vi "LVJSON Dump.vi"(4 "PPIsValue? (F)":bool, 6 "PPIndent (0)":i32, 8 "error in (no error)":errorcluster, 10 "Pretty Print? (F)":bool, 11 "Root Element in":T1) -> (0 "error out":errorcluster, 2 "Key":string, 3 "JSON out":string)   [LabVIEW 2018, in "labview_json.lvlib"]
uses:
  labview_json.lvlib
  Element Type.ctl
  Element.ctl
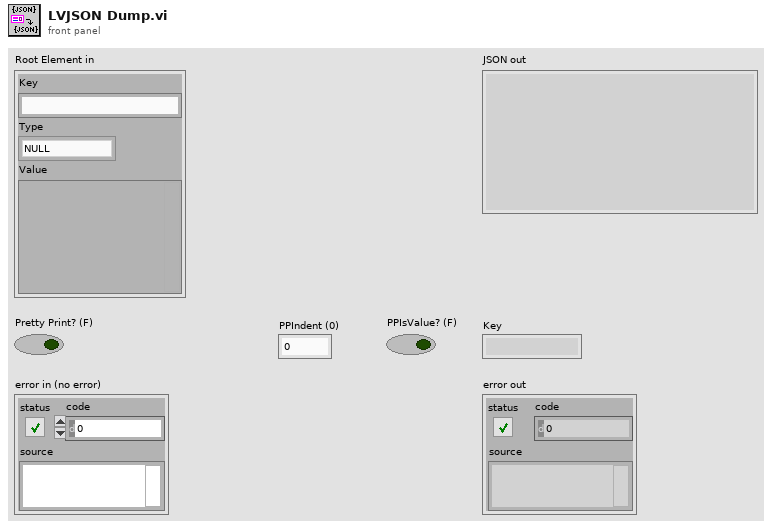
[diagram p1: front panel]
types:
  T1 = typedef "labview_json.lvlib/Element.ctl" = cluster{"Key":string, "Type":T2, "Value":variant}
  T2 = typedef "labview_json.lvlib/Element Type.ctl" = enum8{"NULL", "BOOL", "INT", "UINT", "FLOAT", "STRING", "ARRAY", "OBJECT", "SKIP"}
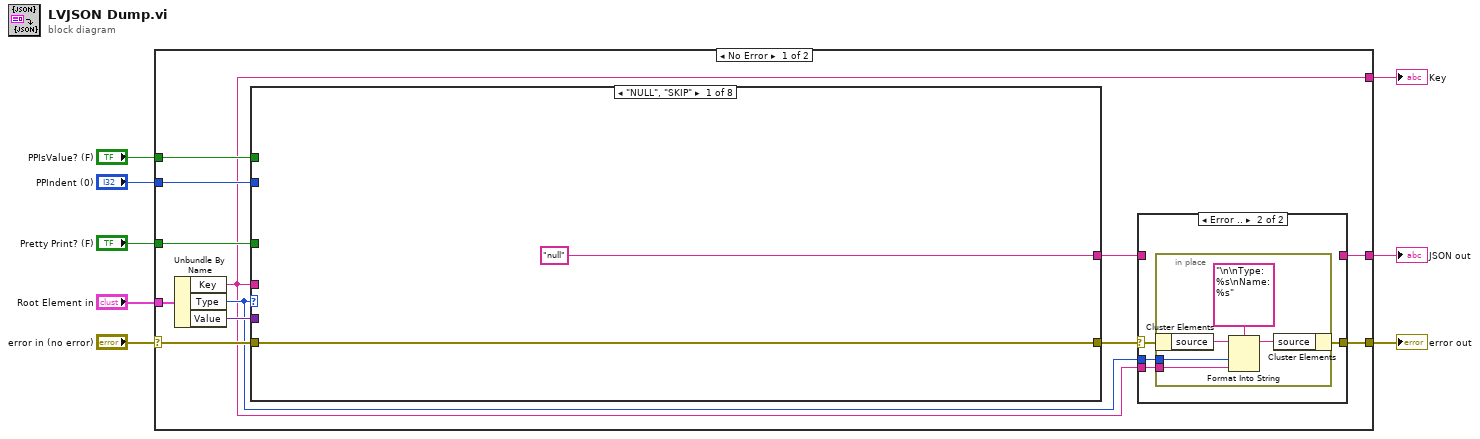
[diagram p0: block diagram]
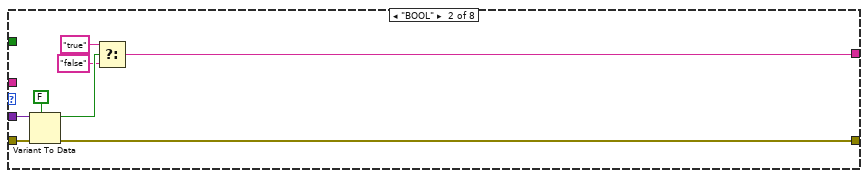
[diagram p2: hidden frame]
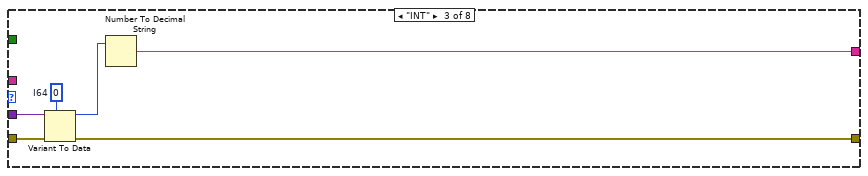
[diagram p3: hidden frame]
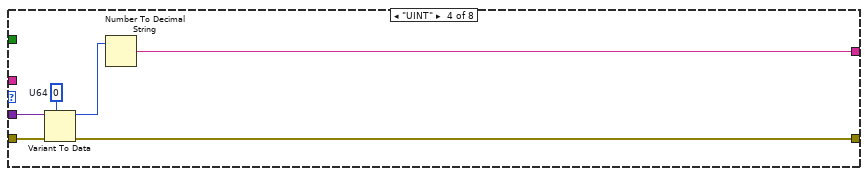
[diagram p4: hidden frame]
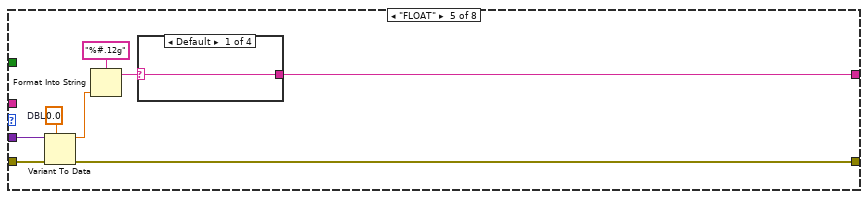
[diagram p5: hidden frame]
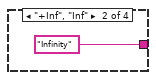
[diagram p6: hidden frame]
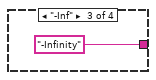
[diagram p7: hidden frame]
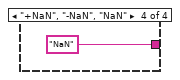
[diagram p8: hidden frame]
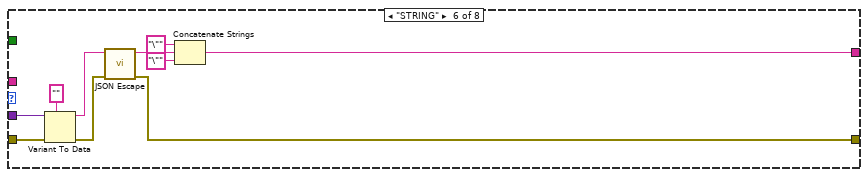
[diagram p9: hidden frame]
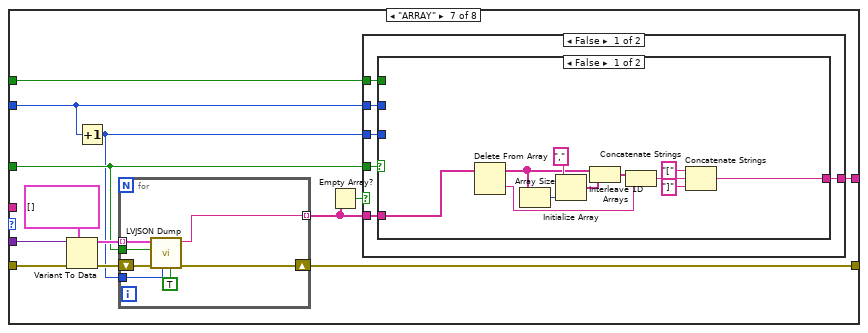
[diagram p10: hidden frame]
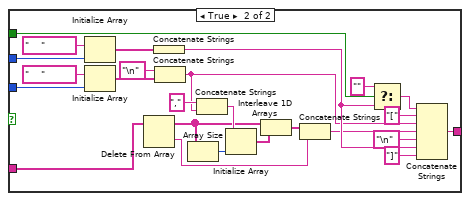
[diagram p11: hidden frame]
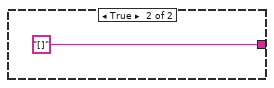
[diagram p12: hidden frame]
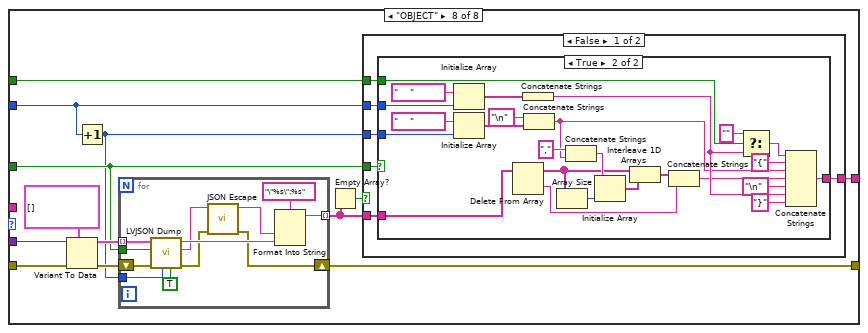
[diagram p13: hidden frame]
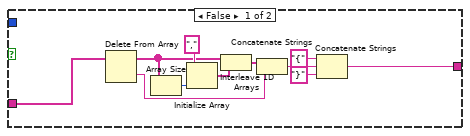
[diagram p14: hidden frame]
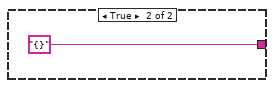
[diagram p15: hidden frame]
diagram:
  n1 = case shown="No Error" "error in (no error)" {
    selector: "error in (no error)" -> [w18 w207]
    tunnel: "Root Element in" -> [w20 _]
    tunnel: [w12 _] -> w7
    tunnel: [w11 w207] -> w5
    tunnel: [w10 _] -> w4
    tunnel: "Pretty Print? (F)" -> [w17 _]
    tunnel: "PPIndent (0)" -> [w16 _]
    tunnel: "PPIsValue? (F)" -> [w15 _]
    frame No Error {
      n2 = Unbundle By Name(w20) -> ("Key"=w12:string, "Type"=w13:T2, "Value"=w19:variant)
      n3 = case shown="\"NULL\", \"SKIP\"" w13 {
        tunnel: w19 -> [_ w28 w34 w40 w48 w63 w77 w140]
        tunnel: w12 -> [_ _ _ _ _ _ _ _]
        tunnel: w18 -> [w21 w30 w36 w42 w50 w64 w75 w138]
        tunnel: [w21 w29 w35 w41 w49 w55 w73 w136] -> w14
        tunnel: ["null" w23 w31 w37 w43 w59 w71 w134] -> w9
        tunnel: w17 -> [_ _ _ _ _ _ w70 w133]
        tunnel: w16 -> [_ _ _ _ _ _ w68 w131]
        tunnel: w15 -> [_ _ _ _ _ _ w69 w132]
        frame "NULL", "SKIP" {
        }
        frame "BOOL" {
          n4 = Variant To Data(error in=w30, type=FALSE, Variant=w28) -> (data=w26:bool, error out=w29:errorcluster)
          n5 = Select(t="true", s=w26, f="false") -> (s? t:f=w23:string)
        }
        frame "INT" {
          w33 = i64 0  # I64
          n6 = Variant To Data(error in=w36, type=w33, Variant=w34) -> (data=w32:i64, error out=w35:errorcluster)
          n7 = Number To Decimal String(number=w32) -> (decimal integer string=w31:string)  [unwired: 1 in]
        }
        frame "UINT" {
          w39 = u64 0  # U64
          n8 = Variant To Data(error in=w42, type=w39, Variant=w40) -> (data=w38:u64, error out=w41:errorcluster)
          n9 = Number To Decimal String(number=w38) -> (decimal integer string=w37:string)  [unwired: 1 in]
        }
        frame "FLOAT" {
          w47 = 0.0  # DBL
          n10 = Variant To Data(error in=w50, type=w47, Variant=w48) -> (data=w46:dbl, error out=w49:errorcluster)
          n11 = Format Into String(format string="%#.12g", w46) -> (resulting string=w44:string)  [unwired: 2 in, 1 out]
          n12 = case shown="Default" w44 {
            selector: w44 -> [w51 _ _ _]
            tunnel: [w51 "Infinity" "-Infinity" "NaN"] -> w43
            frame Default {
            }
            frame "+Inf", "Inf" {
            }
            frame "-Inf" {
            }
            frame "+NaN", "-NaN", "NaN" {
            }
          }
        }
        frame "STRING" {
          n13 = Variant To Data(error in=w64, type="", Variant=w63) -> (data=w61:string, error out=w56:errorcluster)
          n14 = call "JSON Escape.vi"("error in (no error)"=w56, "String"=w61) -> ("error out"=w55:errorcluster, "Escaped String"=w60:string)  [unwired: 7 in, 1 out]
          n15 = Concatenate Strings("\"" ("string"), w60, "\"" ("string")) -> (w59:string)
        }
        frame "ARRAY" {
          n16 = Variant To Data(error in=w75, type=T1[] [], Variant=w77) -> (data=w72:T1[], error out=w74:errorcluster)
          n17 = Increment(x=w68) -> (x+1=w67:i32)
          n18 = for {
            tunnel: w72 -> [w125] mode=indexing
            shift-right: [w126] -> w73
            shift-left: w74 -> [w127]
            tunnel: [w121] -> w66 mode=indexing
            tunnel: w70 -> [w124]
            tunnel: w67 -> [w123]
            n19 = call "LVJSON Dump.vi"("PPIsValue? (F)"=TRUE ("Pretty Print Is Value? (F)"), "PPIndent (0)"=w123, "error in (no error)"=w127, "Pretty Print? (F)"=w124, "Root Element in"=w125) -> ("error out"=w126:errorcluster, "JSON out"=w121:string)  [unwired: 4 in, 1 out]
          }
          n20 = Empty Array?(array=w66) -> (empty?=w65:bool)
          n21 = case shown="False" w65 {
            tunnel: [w83 "[]"] -> w71
            tunnel: w70 -> [w82 _]
            tunnel: w69 -> [w81 _]
            tunnel: w68 -> [w80 _]
            tunnel: w67 -> [w79 _]
            tunnel: w66 -> [w78 _]
            frame False {
              n22 = case shown="False" w82 {
                tunnel: w78 -> [w94 w100]
                tunnel: [w90 w96] -> w83
                tunnel: w81 -> [_ w98]
                tunnel: w80 -> [_ w99]
                tunnel: w79 -> [_ w97]
                frame False {
                  n23 = Delete From Array(array=w94) -> (deleted portion=w84:string, array with subset deleted=w87:string[])  [unwired: 2 in]
                  n24 = Array Size(array=w87) -> (size(s)=w89:i32)
                  n25 = Initialize Array(",", w89) -> (w86:string[])
                  n26 = Interleave 1D Arrays(w87, w86) -> (w85:string[])
                  n27 = Concatenate Strings(w85, w84) -> (w91:string)
                  n28 = Concatenate Strings("[" ("string"), w91, "]" ("string")) -> (w90:string)
                }
                frame True {
                  n29 = Initialize Array("    " ("element"), w99) -> (w117:string[])
                  n30 = Initialize Array("    " ("element"), w97) -> (w113:string[])
                  n31 = Delete From Array(array=w100) -> (deleted portion=w115:string, array with subset deleted=w110:string[])  [unwired: 2 in]
                  n32 = Concatenate Strings(w117) -> (w119:string)
                  n33 = Concatenate Strings("\n" ("element"), w113) -> (w95:string)
                  n34 = Array Size(array=w110) -> (size(s)=w109:i32)
                  n35 = Concatenate Strings("," ("string"), w95) -> (w116:string)
                  n36 = Initialize Array(w116, w109) -> (w111:string[])
                  n37 = Interleave 1D Arrays(w110, w111) -> (w112:string[])
                  n38 = Concatenate Strings(w112, w115) -> (w114:string)
                  n39 = Select(t="", s=w98, f=w119) -> (s? t:f=w118:string)
                  n40 = Concatenate Strings(w118, "[" ("string"), w95, w114, "\n" ("element"), w119, "]" ("string")) -> (w96:string)
                }
              }
            }
            frame True {
            }
          }
        }
        frame "OBJECT" {
          n41 = Variant To Data(error in=w138, type=T1[] [], Variant=w140) -> (data=w135:T1[], error out=w137:errorcluster)
          n42 = Increment(x=w131) -> (x+1=w130:i32)
          n43 = for {
            tunnel: w135 -> [w194] mode=indexing
            shift-right: [w184] -> w136
            shift-left: w137 -> [w195]
            tunnel: [w192] -> w129 mode=indexing
            tunnel: w133 -> [w188]
            tunnel: w130 -> [w187]
            n44 = call "LVJSON Dump.vi"("PPIsValue? (F)"=TRUE ("Pretty Print Is Value? (F)"), "PPIndent (0)"=w187, "error in (no error)"=w195, "Pretty Print? (F)"=w188, "Root Element in"=w194) -> ("error out"=w185:errorcluster, "Key"=w190:string, "JSON out"=w193:string)  [unwired: 4 in]
            n45 = call "JSON Escape.vi"("error in (no error)"=w185, "String"=w190) -> ("error out"=w184:errorcluster, "Escaped String"=w189:string)  [unwired: 7 in, 1 out]
            n46 = Format Into String(format string="\"%s\":%s", w189, w193) -> (resulting string=w192:string)  [unwired: 2 in, 1 out]
          }
          n47 = Empty Array?(array=w129) -> (empty?=w128:bool)
          n48 = case shown="False" w128 {
            tunnel: [w146 "{}"] -> w134
            tunnel: w133 -> [w145 _]
            tunnel: w132 -> [w144 _]
            tunnel: w131 -> [w143 _]
            tunnel: w130 -> [w142 _]
            tunnel: w129 -> [w141 _]
            frame False {
              n49 = case shown="True" w145 {
                tunnel: w141 -> [w157 w163]
                tunnel: [w153 w159] -> w146
                tunnel: w144 -> [_ w161]
                tunnel: w143 -> [_ w162]
                tunnel: w142 -> [_ w160]
                frame False {
                  n50 = Delete From Array(array=w157) -> (deleted portion=w147:string, array with subset deleted=w150:string[])  [unwired: 2 in]
                  n51 = Array Size(array=w150) -> (size(s)=w152:i32)
                  n52 = Initialize Array(",", w152) -> (w149:string[])
                  n53 = Interleave 1D Arrays(w150, w149) -> (w148:string[])
                  n54 = Concatenate Strings(w148, w147) -> (w154:string)
                  n55 = Concatenate Strings("{" ("string"), w154, "}" ("string")) -> (w153:string)
                }
                frame True {
                  n56 = Initialize Array("    " ("element"), w162) -> (w180:string[])
                  n57 = Initialize Array("    " ("element"), w160) -> (w176:string[])
                  n58 = Delete From Array(array=w163) -> (deleted portion=w178:string, array with subset deleted=w173:string[])  [unwired: 2 in]
                  n59 = Concatenate Strings(w180) -> (w182:string)
                  n60 = Concatenate Strings("\n" ("element"), w176) -> (w158:string)
                  n61 = Array Size(array=w173) -> (size(s)=w172:i32)
                  n62 = Concatenate Strings("," ("string"), w158) -> (w179:string)
                  n63 = Initialize Array(w179, w172) -> (w174:string[])
                  n64 = Interleave 1D Arrays(w173, w174) -> (w175:string[])
                  n65 = Concatenate Strings(w175, w178) -> (w177:string)
                  n66 = Select(t="", s=w161, f=w182) -> (s? t:f=w181:string)
                  n67 = Concatenate Strings(w181, "{" ("string"), w158, w177, "\n" ("element"), w182, "}" ("string")) -> (w159:string)
                }
              }
            }
            frame True {
            }
          }
        }
      }
      n68 = case shown="Error .." w14 {
        selector: w14 -> [w197 w201]
        tunnel: [w197 w200] -> w11
        tunnel: w13 -> [_ w199]
        tunnel: w12 -> [_ w198]
        tunnel: [w196 _] -> w10
        tunnel: w9 -> [w196 _]
        frame No Error {
        }
        frame Error {
          n69 = in-place {
            in-place-border: w199 -> [w203]
            in-place-border: w198 -> [w202]
            n70 = in-place-cluster #1(w201) -> ("source"=w206:string)
            n71 = Format Into String(format string="\n\nType: %s\nName: %s", initial string=w206, w203, w202) -> (resulting string=w205:string)  [unwired: 1 in, 1 out]
            n72 = in-place-cluster #1("source"=w205) -> (w200:errorcluster)
          }
        }
      }
    }
    frame Error {
    }
  }
  "JSON out" <- w4
  "error out" <- w5
  "Key" <- w7
